vi "Build Word.vi"() -> ()   [LabVIEW 2020]
uses:
  Parameter Definition.ctl
  Encoding and Decoding/Encoding.ctl
  32-bit Word.lvclass/32-bit Word.ctl
  32-bit Word.lvclass
  ARINC 429.lvclass
  Encoding and Decoding/Encoding and Decoding.lvlib
panel:
  out "parameters values decoded":dbl[](array[numeric])
  in  "parameters definitions":T1[](array[typedef])=[{"start index"=23, "size"=6, "encoding"=enum."BCD", "signed"=FALSE, "scale multiplier"=1.0, "scale offset"=0.0}, {"start index"=18, "size"=5, "encoding"=enum."BCD", "signed"=FALSE, "scale multiplier"=1.0, "scale offset"=0.0}, {"start index"=10, "size"=8, "encoding"=enum."BNR", "signed"=FALSE, "scale multiplier"=1.0, "scale offset"=0.0}]
  in  "parameters values":dbl[](array[numeric])=[23.0, 3.0, 17.0]
  out "32-bit word 2":u32 format="%032b"
  out "error out 2":errorcluster
  in  "label value 2":u8=176 format="%.0o"
  in  "SDI value 2":u8 format="%02b"
  out "parameter value":dbl=nan
  in  "parameter definition":T1={"start index"=10, "size"=19, "encoding"=enum."BNR", "signed"=TRUE, "scale multiplier"=1.0, "scale offset"=0.0}
  in  "data":dbl=-123.0
  in  "SDI value":u8=3 format="%02b"
  in  "label value":u8=134 format="%.0o"
  out "error out":errorcluster
  out "32-bit word":u32 format="%032b"
  # "10010001100011000100010000001101"
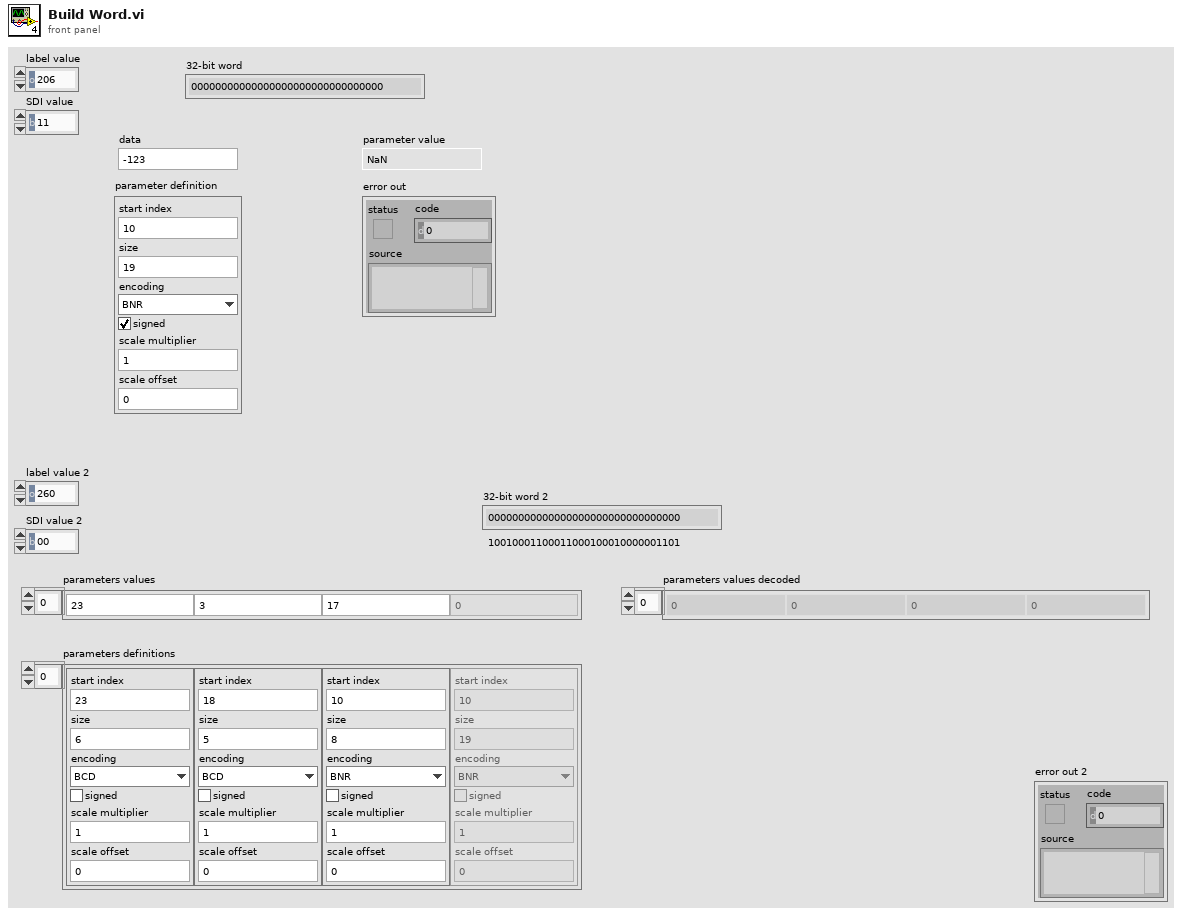
[diagram p1: front panel]
types:
  T1 = typedef "ARINC 429.lvclass/Parameter Definition.ctl" = cluster{"start index":i32, "size":i32, "encoding":T2, "signed":bool, "scale multiplier":dbl, "scale offset":dbl}
  T2 = typedef "Encoding and Decoding.lvlib/Encoding.ctl" = enum16{"BNR", "BCD", "Discrete"}
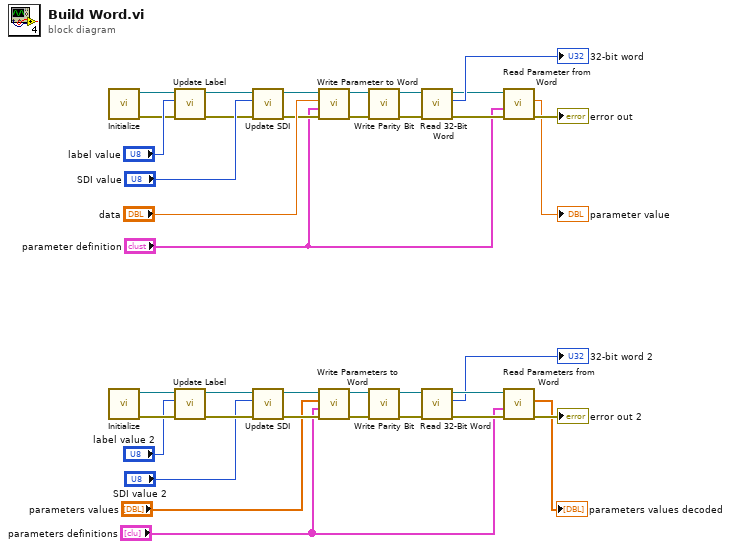
[diagram p0: block diagram]
diagram:
  n1 = call "Initialize.vi"() -> ("error out"=w33:errorcluster, "ARINC 429 (32-bit word)"=w38:refnum<class "32-bit Word.lvclass">)  [unwired: 10 in]
  n2 = call "Initialize.vi"() -> ("error out"=w11:errorcluster, "ARINC 429 (32-bit word)"=w5:refnum<class "32-bit Word.lvclass">)  [unwired: 10 in]
  n3 = call-dynamic "Update Label.vi"("error in"=w33, "label value"="label value", "32-bit word in"=w38) -> ("error out"=w32:errorcluster, "32-bit word out"=w1:refnum<class "32-bit Word.lvclass">)  [unwired: 7 in]
  n4 = call-dynamic "Update Label.vi"("error in"=w11, "label value"="label value 2", "32-bit word in"=w5) -> ("error out"=w12:errorcluster, "32-bit word out"=w9:refnum<class "32-bit Word.lvclass">)  [unwired: 7 in]
  n5 = call-dynamic "Update SDI.vi"("error in"=w32, "SDI value"="SDI value", "32-bit Word in"=w1) -> ("error out"=w28:errorcluster, "32-bit Word out"=w29:refnum<class "32-bit Word.lvclass">)  [unwired: 7 in]
  n6 = call-dynamic "Update SDI.vi"("error in"=w12, "SDI value"="SDI value 2", "32-bit Word in"=w9) -> ("error out"=w15:errorcluster, "32-bit Word out"=w14:refnum<class "32-bit Word.lvclass">)  [unwired: 7 in]
  n7 = call-dynamic "Write Parameter to Word.vi"("error in"=w28, "parameter definition"="parameter definition", "data"="data", "32-bit Word in"=w29) -> ("error out"=w27:errorcluster, "32-bit Word out"=w26:refnum<class "32-bit Word.lvclass">)  [unwired: 6 in]
  n8 = call-dynamic "Write Parameters to Word.vi"("error in"=w15, "parameters definitions"="parameters definitions", "parameters values"="parameters values", "32-bit Word in"=w14) -> ("error out"=w16:errorcluster, "32-bit Word out"=w17:refnum<class "32-bit Word.lvclass">)  [unwired: 6 in]
  n9 = call-dynamic "Write Parity Bit.vi"("error in"=w27, "32-bit word in"=w26) -> ("error out"=w31:errorcluster, "32-bit word out"=w34:refnum<class "32-bit Word.lvclass">)  [unwired: 8 in]
  n10 = call-dynamic "Write Parity Bit.vi"("error in"=w16, "32-bit word in"=w17) -> ("error out"=w13:errorcluster, "32-bit word out"=w10:refnum<class "32-bit Word.lvclass">)  [unwired: 8 in]
  n11 = call "Read 32-Bit Word.vi"("error in (no error)"=w31, "32-bit Word in"=w34) -> ("error out"=w24:errorcluster, "32-bit word"=→"32-bit word":u32, "32-bit Word out"=w25:refnum<class "32-bit Word.lvclass">)  [unwired: 7 in]
  n12 = call "Read 32-Bit Word.vi"("error in (no error)"=w13, "32-bit Word in"=w10) -> ("error out"=w19:errorcluster, "32-bit word"=→"32-bit word 2":u32, "32-bit Word out"=w18:refnum<class "32-bit Word.lvclass">)  [unwired: 7 in]
  n13 = call-dynamic "Read Parameter from Word.vi"("error in"=w24, "parameter definition"="parameter definition", "32-bit Word in"=w25) -> ("error out"=→"error out":errorcluster, "parameter value"=→"parameter value":dbl)  [unwired: 6 in, 1 out]
  n14 = call-dynamic "Read Parameters from Word.vi"("error in"=w19, "parameters definitions"="parameters definitions", "32-bit Word in"=w18) -> ("error out"=→"error out 2":errorcluster, "parameters values"=→"parameters values decoded":dbl[])  [unwired: 6 in, 1 out]
